vi "Target.vi"() -> ()   [LabVIEW 2017]
uses:
  <vilib>/myRIO/Instrument Drivers/Utilities/Utilities.lvlib
  <vilib>/Platform/TimedLoop/XDataNode/XDataNode.xnode
  <vilib>/Platform/TimedLoop/XDataNode/nitl_modes.ctl
  <vilib>/Platform/TimedLoop/XDataNode/XDNodeRunTimeDep.lvlib
  <vilib>/Platform/TimedLoop/XDataNode/wakeup.ctl
  <vilib>/Platform/TimedLoop/XDataNode/timing_clust.ctl
  <vilib>/myRIO/Express VI/Onboard IO/PWM/PWM Express VI.xnode
  <vilib>/myRIO/Instrument Drivers/Onboard IO/PWM/vis/Set Duty Cycle and Frequency.vi
  <vilib>/myRIO/Instrument Drivers/Onboard IO/PWM/PWM.lvlib
  <vilib>/myRIO/Instrument Drivers/Onboard IO/PWM/typedefs/PWM Configuration.ctl
  <vilib>/myRIO/Common/Instrument Driver Framework/myRIO v1.0/PWM/typedefs/PWM Channels Enum.ctl
  <vilib>/myRIO/Common/Instrument Driver Framework/Utilities/typedefs/Generic FPGA Reference.ctl
  <vilib>/myRIO/Common/Instrument Driver Framework/Utilities/typedefs/myRIO v1.0 Reference.ctl
  <vilib>/myRIO/Common/Instrument Driver Framework/Utilities/typedefs/Hardware Version Enum.ctl
  <vilib>/myRIO/Common/Instrument Driver Framework/Utilities/typedefs/myRIO Generic Hardware Reference.ctl
  <vilib>/myRIO/Instrument Drivers/Onboard IO/PWM/typedefs/PWM Reference.ctl
  <vilib>/myRIO/Instrument Drivers/Onboard IO/PWM/vis/myRIO PWM Open.xnode
  <vilib>/myRIO/Common/Instrument Driver Framework/Utilities/vis/Is FPGA Ref Available.vi
  <vilib>/myRIO/Common/Instrument Driver Framework/myRIO v1.0/PWM/vis/myRIO v1.1 Open PWM.vi
  <vilib>/userdefined/High Color/nirio_resource_hc.ctl
panel:
  out "Pump Duty Cycle":dbl=0.5
  out "Iteration Duration":i64
  in  "Pause":bool
  in  "stop":bool
  out "Target Running":bool
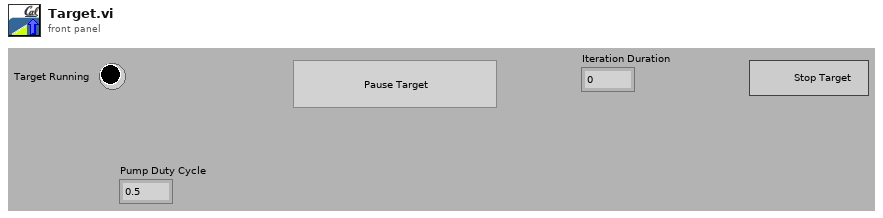
[diagram p1: front panel]
types:
  T1 = typedef "XDNodeRunTimeDep.lvlib/timing_clust.ctl" = cluster{"Expected End [f-1]":u64, "Actual End [f-1]":u64, "Finished Late? [f-1]":bool, "Expected End [i-1]":u64, "Actual End [i-1]":u64, "Finished Late? [i-1]":bool, "Expected Start [i]":u64, "Actual Start [i]":u64, "Expected Start [f]":u64, "Actual Start [f]":u64, "Source Name":string, "Structure Name":string, "Period":i64, "Deadline":i64, "Offset":i64, "Start":i64, "Priority":i32, "Timeout":i32, "Mode":T2, "Wakeup Reason":T3, "Error":errorcluster, "Source Type":string, "Secondary Source Type":string, "Global End Time":u64, "Global Start Time":u64, "Frame Duration":u64, "Iteration Duration":u64, "Assigned CPU":i32, "I/O Scan Engine Mode":u32}
  T2 = typedef "XDNodeRunTimeDep.lvlib/nitl_modes.ctl" = enum32{"No Change", "Process missed periods, maintain original phase", "Discard missed periods, maintain original phase", "Process missed periods, ignore original phase", "Discard missed periods, ignore original phase"}
  T3 = typedef "XDNodeRunTimeDep.lvlib/wakeup.ctl" = enum32{"Normal", "Aborted", "Asynchronous wakeup", "Timing source error", "Timed loop error", "Timeout"}
  T4 = typedef "PWM.lvlib/PWM Reference.ctl" = cluster{"myRIO Reference":T5, "PWM Channels Enum":T9, "PWM Configuration":T10}
  T5 = typedef "myRIO Generic Hardware Reference.ctl" = cluster{"myRIO Model":T6, "myRIO Hardware Reference":T7}
  T6 = typedef "Hardware Version Enum.ctl" = enum16{"Unknown", "myRIO-1900", "myRIO-1950", "roboRIO", "NI ELVIS RIO CM"}
  T7 = typedef "myRIO v1.0 Reference.ctl" = cluster{"Generic FPGA Reference":T8, "Allow multiple opens":bool}
  T8 = typedef "Generic FPGA Reference.ctl" = refnum<k20>
  T9 = typedef "PWM Channels Enum.ctl" = enum16{"Not Connected", "C/PWM0", "C/PWM1", "A/PWM0", "A/PWM1", "A/PWM2", "B/PWM0", "B/PWM1", "B/PWM2", "PWM/PWM0", "PWM/PWM1", "PWM/PWM2", "PWM/PWM3", "PWM/PWM4", "PWM/PWM5", "PWM/PWM6", "PWM/PWM7", "PWM/PWM8", "PWM/PWM9"}
  T10 = typedef "PWM.lvlib/PWM Configuration.ctl" = cluster{"Frequency":dbl, "Duty Cycle":dbl}
  T11 = typedef "nirio_resource_hc.ctl" = tag
  T12 = cluster{"X":dbl, "Y":dbl, "h_ratio":dbl, "Match?":bool}
  T13 = typedef "Outputs.ctl" = cluster{"x position":dbl, "y position":dbl, "Pump Duty Cycle":dbl, "Y Direction":bool, "Stop Servos":bool}
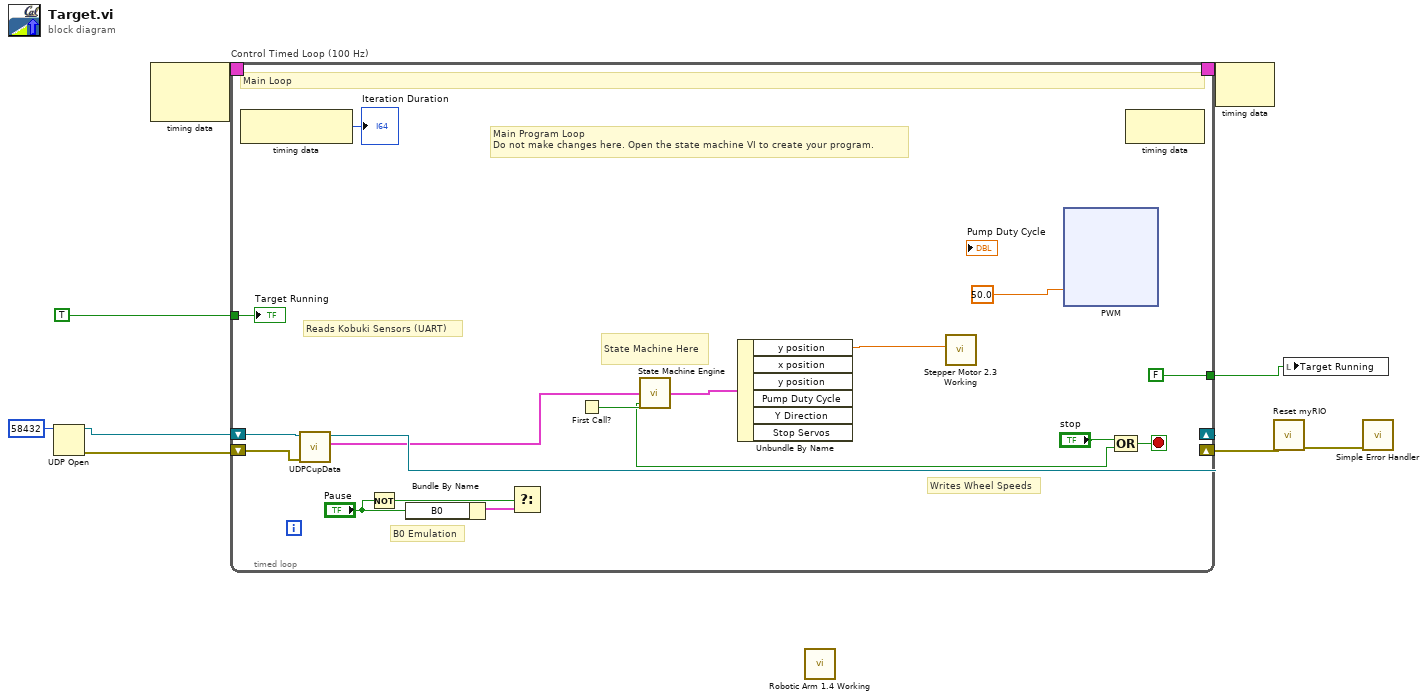
[diagram p0: block diagram]
diagram:
  n1 = UDP Open(11:u16 58432 ("port")) -> (port=w2:refnum<k16>, 0:w3:errorcluster)  [unwired: 4 in, 1 out]
  n2 = node-c288() -> (w6:T1)  [unwired: 2 in]
  n3 = timed-loop "Control Timed Loop (100 Hz)" {
    shift-right: [_] -> w1
    shift-left: w3 -> [w15]
    tunnel: TRUE ("stop") -> [w24]
    tunnel: [FALSE ("stop")] -> w8
    timing: w6 -> [_]
    timing-out: [_] -> w5
    shift-right: [w12] -> _
    shift-left: w2 -> [w14]
    stop <- w26 stop-if-true
    # "B0 Emulation"
    # "Main Program Loop\nDo not make changes here. Open the state machine VI to create your program."
    # "Writes Wheel Speeds"
    # "Reads Kobuki Sensors (UART)"
    # "State Machine Here"
    # "Main Loop"
    n4 = node-c288() -> (→"Iteration Duration":i64)  [unwired: 1 in]
    n5 = call "UDPCupData.vi"("error in (no error)"=w15, "UDP Network Connection in"=w14) -> ("Cup Data"=w11:T12, "UDP Network Connection out"=w12:refnum<k16>)  [unwired: 7 in, 1 out]
    n6 = Not(x="Pause") -> (.not. x?=w18:bool)
    n7 = Bundle By Name("B0"="Pause") -> (w20:cluster{})  [unwired: 1 in]
    n8 = Select(s=w18, f=w20) -> ()  [unwired: 1 in, 1 out]
    n9 = First Call?() -> (First Call?: T/F=w22:bool)
    n10 = call "State Machine Engine.vi"("Init?"=w22, "Inputs"=w11) -> ("Terminated?"=w21:bool, "Outputs"=w23:T13)  [unwired: 1 in, 1 out]
    n11 = Unbundle By Name(w23) -> ("y position"=w13:dbl)  [unwired: 5 out]
    n12 = call "Stepper Motor 2.3 Working.vi"("y (inches)"=w13) -> ()  [unwired: 11 in]
    n13 = xnode "PWM"("Frequency [Hz]"=50.0) -> ()  [unwired: 2 in, 1 out]
    n14 = Compound Arithmetic op=OR("stop", w21) -> (w26:bool)
    n15 = node-c288() -> ()  [unwired: 1 in, 1 out]
    "Target Running" <- w24
  }
  n16 = call "Robotic Arm 1.4 Working.vi"() -> ()  [unwired: 12 in]
  n17 = node-c288(w5) -> ()  [unwired: 1 out]
  n18 = call <vilib>:"Reset myRIO.vi"("error in (no error)"=w1) -> ("error out"=w7:errorcluster)  [unwired: 10 in]
  n19 = local write "Target Running"(w8) -> ()
  n20 = call <vilib>:"Simple Error Handler.vi"("error in (no error)"=w7) -> ()  [unwired: 4 in, 5 out]
